vi "cosmeticPIP.vi"(8 "error in (no error)":errorcluster) -> (0 "error out":errorcluster, 3 "COSMETIC-3, 4":string)   [LabVIEW 2018]
uses:
  Global_1259.vi
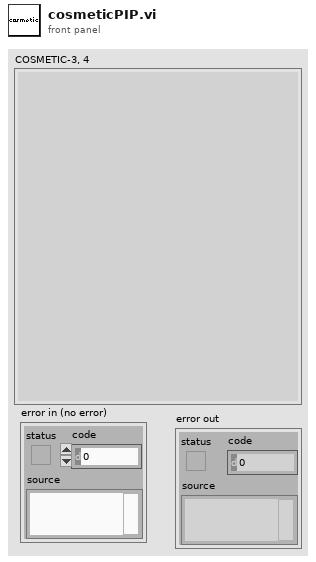
[diagram p1: front panel]
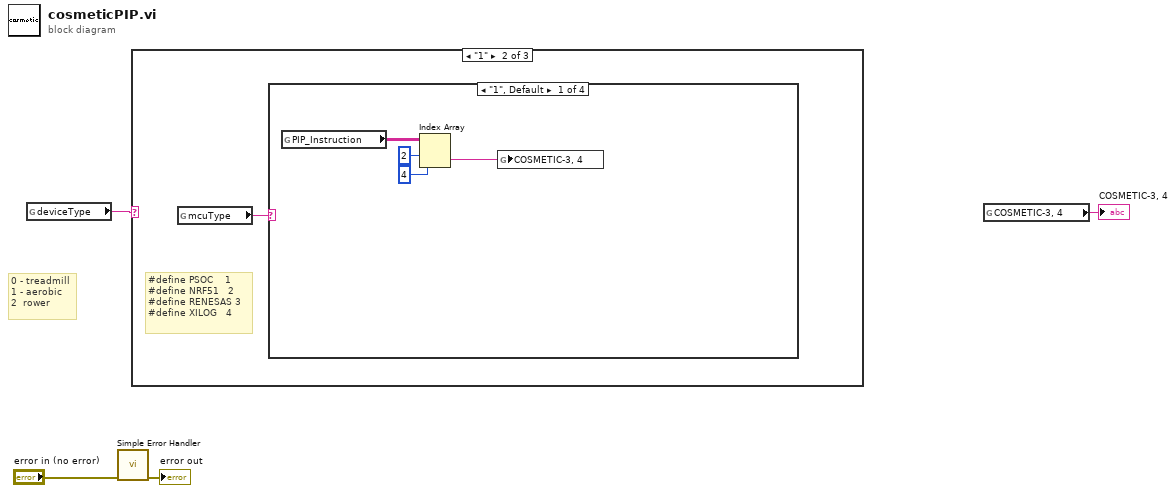
[diagram p0: block diagram]
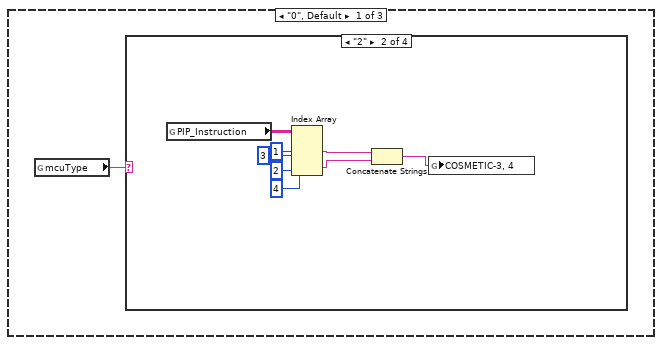
[diagram p2: hidden frame]
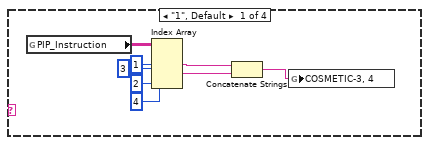
[diagram p3: hidden frame]
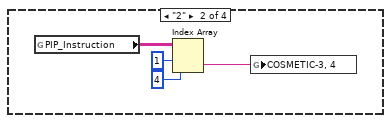
[diagram p6: hidden frame]
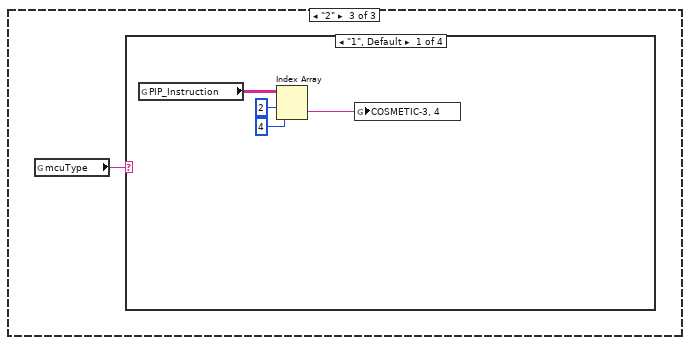
[diagram p9: hidden frame]
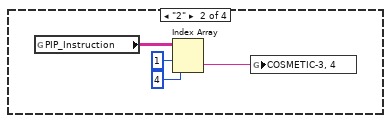
[diagram p10: hidden frame]
diagram:
  # "0 - treadmill\n1 - aerobic\n2  rower"
  n1 = global read "Global_1259.vi" "deviceType"() -> (w2:string)
  n2 = call <vilib>:"Simple Error Handler.vi"("error in (no error)"="error in (no error)") -> ("error out"=→"error out":errorcluster)  [unwired: 4 in, 4 out]
  n3 = case shown="\"1\"" w2 {
    frame "0", Default {
      n4 = global read "Global_1259.vi" "mcuType"() -> (w5:string)
      n5 = case shown="\"2\"" w5 {
        frame "1", Default {
          n6 = global read "Global_1259.vi" "PIP_Instruction"() -> (w13:string[][])
          n7 = Index Array(array=w13, index (row) #1=1 ("index (row)"), index (col) #1=3 ("disabled index (col)"), index (row) #2=2 ("index (row)"), index (col) #2=4 ("disabled index (col)")) -> (element #1=w8:string, element #2=w6:string)
          n8 = Concatenate Strings(w8, w6) -> (w7:string)
          n9 = global write "Global_1259.vi" "COSMETIC-3, 4"(w7) -> ()
        }
        frame "2" {
          n10 = global read "Global_1259.vi" "PIP_Instruction"() -> (w21:string[][])
          n11 = Index Array(array=w21, index (row) #1=1 ("index (row)"), index (col) #1=3 ("disabled index (col)"), index (row) #2=2 ("index (row)"), index (col) #2=4 ("disabled index (col)")) -> (element #1=w16:string, element #2=w14:string)
          n12 = Concatenate Strings(w16, w14) -> (w15:string)
          n13 = global write "Global_1259.vi" "COSMETIC-3, 4"(w15) -> ()
        }
        frame "3" {
        }
        frame "4" {
        }
      }
    }
    frame "1" {
      # "#define PSOC    1\n#define NRF51   2\n#define RENESAS 3\n#define XILOG   4"
      n14 = global read "Global_1259.vi" "mcuType"() -> (w22:string)
      n15 = case shown="\"1\", Default" w22 {
        frame "1", Default {
          n16 = global read "Global_1259.vi" "PIP_Instruction"() -> (w26:string[][])
          n17 = Index Array(array=w26, index (row)=2, index (col)=4 ("disabled index (col)")) -> (element=w23:string)
          n18 = global write "Global_1259.vi" "COSMETIC-3, 4"(w23) -> ()
        }
        frame "2" {
          n19 = global read "Global_1259.vi" "PIP_Instruction"() -> (w30:string[][])
          n20 = Index Array(array=w30, index (row)=1, index (col)=4 ("disabled index (col)")) -> (element=w27:string)
          n21 = global write "Global_1259.vi" "COSMETIC-3, 4"(w27) -> ()
        }
        frame "3" {
        }
        frame "4" {
        }
      }
    }
    frame "2" {
      n22 = global read "Global_1259.vi" "mcuType"() -> (w31:string)
      n23 = case shown="\"1\", Default" w31 {
        frame "1", Default {
          n24 = global read "Global_1259.vi" "PIP_Instruction"() -> (w35:string[][])
          n25 = Index Array(array=w35, index (row)=2, index (col)=4 ("disabled index (col)")) -> (element=w32:string)
          n26 = global write "Global_1259.vi" "COSMETIC-3, 4"(w32) -> ()
        }
        frame "2" {
          n27 = global read "Global_1259.vi" "PIP_Instruction"() -> (w39:string[][])
          n28 = Index Array(array=w39, index (row)=1, index (col)=4 ("disabled index (col)")) -> (element=w36:string)
          n29 = global write "Global_1259.vi" "COSMETIC-3, 4"(w36) -> ()
        }
        frame "3" {
        }
        frame "4" {
        }
      }
    }
  }
  n30 = global read "Global_1259.vi" "COSMETIC-3, 4"() -> (→"COSMETIC-3, 4":string)
